vi "fileName.vi"() -> ()   [LabVIEW 2017]
panel:
  in  "FileName":string
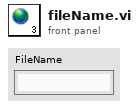
[diagram p1: front panel]
diagram:
